vi "Init.vi"(8 "error in (no error)":errorcluster, 11 "Object (subject) in":refnum<class "Object (subject).lvclass">) -> (0 "error out":errorcluster, 3 "Object (subject) out":refnum<class "Object (subject).lvclass">)   [LabVIEW 2014, in "Object (subject).lvclass"]
uses:
  Object (subject).lvclass
  Object (subject).lvclass/Object (subject).ctl
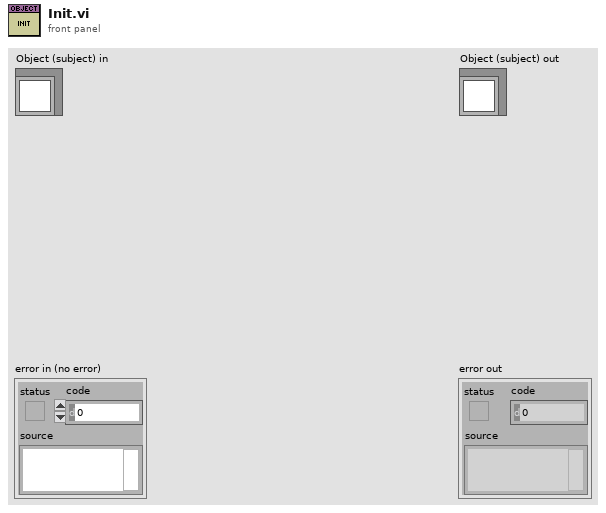
[diagram p1: front panel]
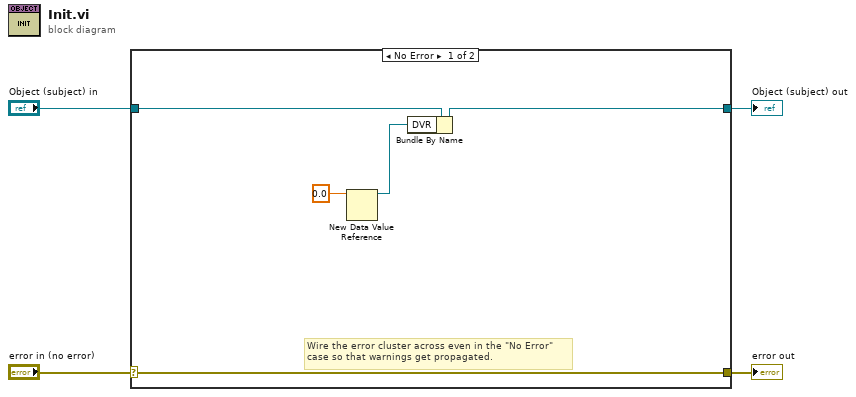
[diagram p0: block diagram]
diagram:
  n1 = case shown="No Error" "error in (no error)" {
    selector: "error in (no error)" -> [w8 w11]
    tunnel: [w8 w11] -> w3
    tunnel: [w6 w10] -> w1
    tunnel: "Object (subject) in" -> [w9 w10]
    frame No Error {
      # "Wire the error cluster across even in the \"No Error\"\ncase so that warnings get propagated."
      n2 = New Data Value Reference(data value=0.0) -> (data value reference=w5:refnum<data-value>)  [unwired: 1 in, 1 out]
      n3 = Bundle By Name(cluster=w9, "DVR"=w5) -> (w6:refnum<class "Object (subject).lvclass">)
    }
    frame Error {
    }
  }
  "error out" <- w3
  "Object (subject) out" <- w1
